vi "Calc Cmd Chans.vi"(8 "error in (no error)":errorcluster, 11 "Calculation in":refnum<class "Calculation.lvclass">) -> (0 "error out":errorcluster, 1 "Numeric Cmd Chans":string[](array[string]), 2 "Digital Cmd Chans":string[](array[string]), 3 "Calculation out":refnum<class "Calculation.lvclass">)   [LabVIEW 2020, in "VolatusCalcs.lvlib" / "Calculation.lvclass"]
uses:
  Calculation.lvclass
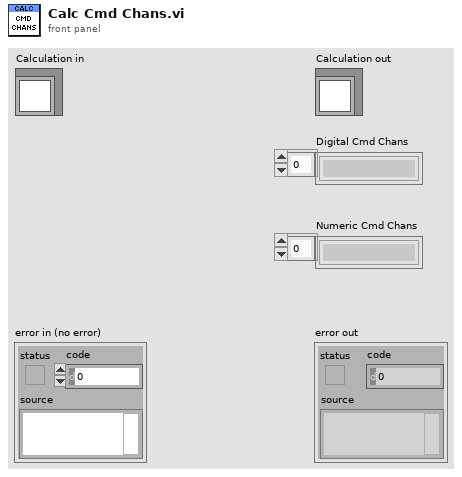
[diagram p1: front panel]
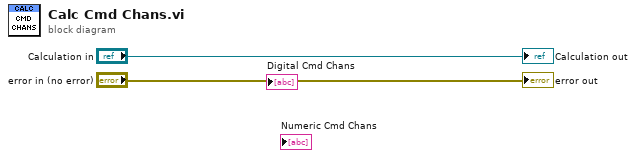
[diagram p0: block diagram]
diagram:
  "error out" <- "error in (no error)"
  "Calculation out" <- "Calculation in"
